vi "Get Channel Glyph Index.vi"(11 "Channel Type":T1) -> (3 "Glyph Index":i32)   [LabVIEW 2015, in "Shared Variable Custom Device.lvlib"]
uses:
  Shared Variable Custom Device.lvlib
  <vilib>/Utility/VariantDataType/Type.ctl
  Shared/Shared Variable Globals.vi
  <vilib>/Utility/VariantDataType/VariantType.lvlib
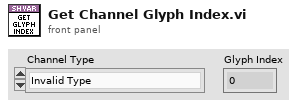
[diagram p1: front panel]
types:
  T1 = typedef "VariantType.lvlib/Type.ctl" = enum8{"Invalid Type", "Void", "I8", "I16", "I32", "I64", "U8", "U16", "U32", "U64", "Single Float", "Double Float", "Extended Float", "Single Complex", "Double Complex", "Extended Complex", "Enum U8", "Enum U16", "Enum U32", "Enum U64", "Single Float With Unit", "Double Float With Unit", "Extended Float With Unit", "Single Complex with Unit", "Double Complex with Unit", "Extended Complex with Unit", "Boolean", "String", "Path", "Picture", "Tag", "Array", "Cluster", "Variant", "LV Variant", "Waveform", "Timestamp", "Digital Waveform", "Digital Data", "ExpressData", "Refnum", "External Data", "VI", "Poly VI", "LabVIEW Class Instance", "Fixed Point"}
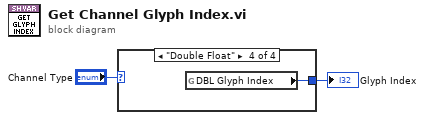
[diagram p0: block diagram]
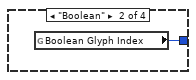
[diagram p3: hidden frame]
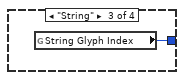
[diagram p4: hidden frame]
diagram:
  n1 = case shown="\"Double Float\"" "Channel Type" {
    tunnel: [_ w3 w4 w5] -> w1
    frame Default {
    }
    frame "Boolean" {
      n2 = global read "Shared Variable Globals.vi" "Boolean Glyph Index"() -> (w3:i32)
    }
    frame "String" {
      n3 = global read "Shared Variable Globals.vi" "String Glyph Index"() -> (w4:i32)
    }
    frame "Double Float" {
      n4 = global read "Shared Variable Globals.vi" "DBL Glyph Index"() -> (w5:i32)
    }
  }
  "Glyph Index" <- w1
